vi "curvature-cator.vi"(4 "number of grid points":i32=300, 5 "decimation threshold":i32=3, 6 "first time":bool, 7 "size":i32=1, 8 "scale factor":dbl=3.0, 9 "wavepacket in":T2={"R"=0.5, "wave number"=22.0, "delta k"=7.0, "radii vector"=[], "radial section"=[], "wave vector"=22.0, "wavepacket is"=TRUE} {"delta k" format="%#_3f"; "wave number" format="%#_3f"; "R" format="%#_3f"}, 10 "z array in":cdb[](array[numeric]), 11 "omega array in":dbl[](array[numeric])) -> (1 "4 corners out":T1={"z (-pi/2)"=-1.0311345636926572+0.5736824521422934i, "z(inf)"=-0.5200164984937075+1.0975277942502903i, "z (pi/2)"=-1.0311345636926572+0.5736824521422934i, "z center"=-0.5136528600391839+0.580046090596817i, "z(0)"=-0.5200164984937075+1.0975277942502903i, "radius"=-1.0311345636926572}, 2 "spot size":dbl, 3 "spot center":cdb)   [LabVIEW 2018]
uses:
  wavepacket.ctl
  circle corners.ctl
  complex region.ctl
  <vilib>/Analysis/baseanly.llb/Median.vi
  <vilib>/Analysis/baseanly.llb/Mean.vi
  <vilib>/Analysis/baseanly.llb/Mean (DBL).vi
panel:
  out "mean":cdb
  in  "number":cdb
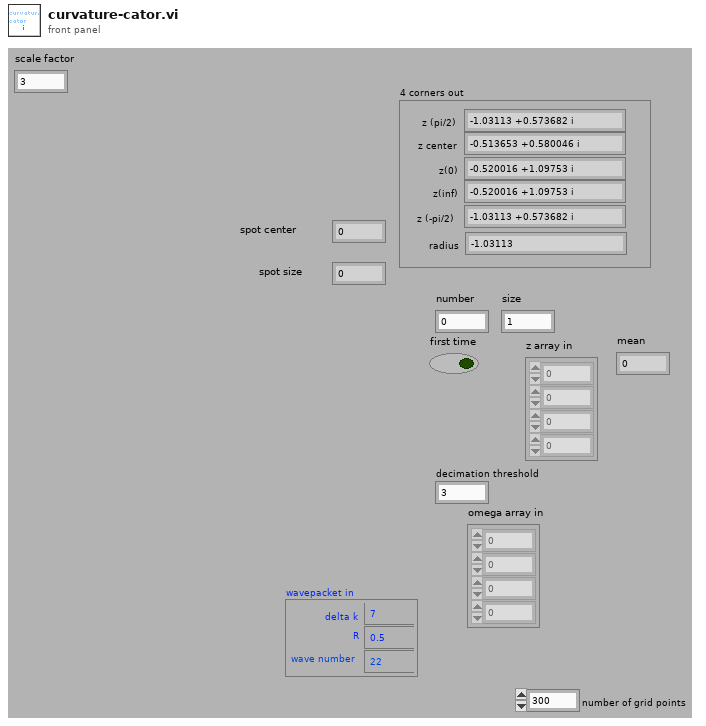
[diagram p1: front panel]
types:
  T1 = typedef "circle corners.ctl" = cluster{"z (-pi/2)":cdb, "z(inf)":cdb, "z (pi/2)":cdb, "z center":cdb, "z(0)":cdb, "radius":dbl}
  T2 = typedef "wavepacket.ctl" = cluster{"R":dbl, "wave number":dbl, "delta k":dbl, "radii vector":dbl[], "radial section":cdb[], "wave vector":dbl, "wavepacket is":bool}
  T3 = typedef "complex region.ctl" = cluster{"max re":dbl, "min re":dbl, "max im":dbl, "min im":dbl, "delta re":dbl, "delta im":dbl, "center re":dbl, "delta  z":cdb, "center im":dbl, "center z":cdb, "d im":dbl, "d re":dbl, "d z":cdb}
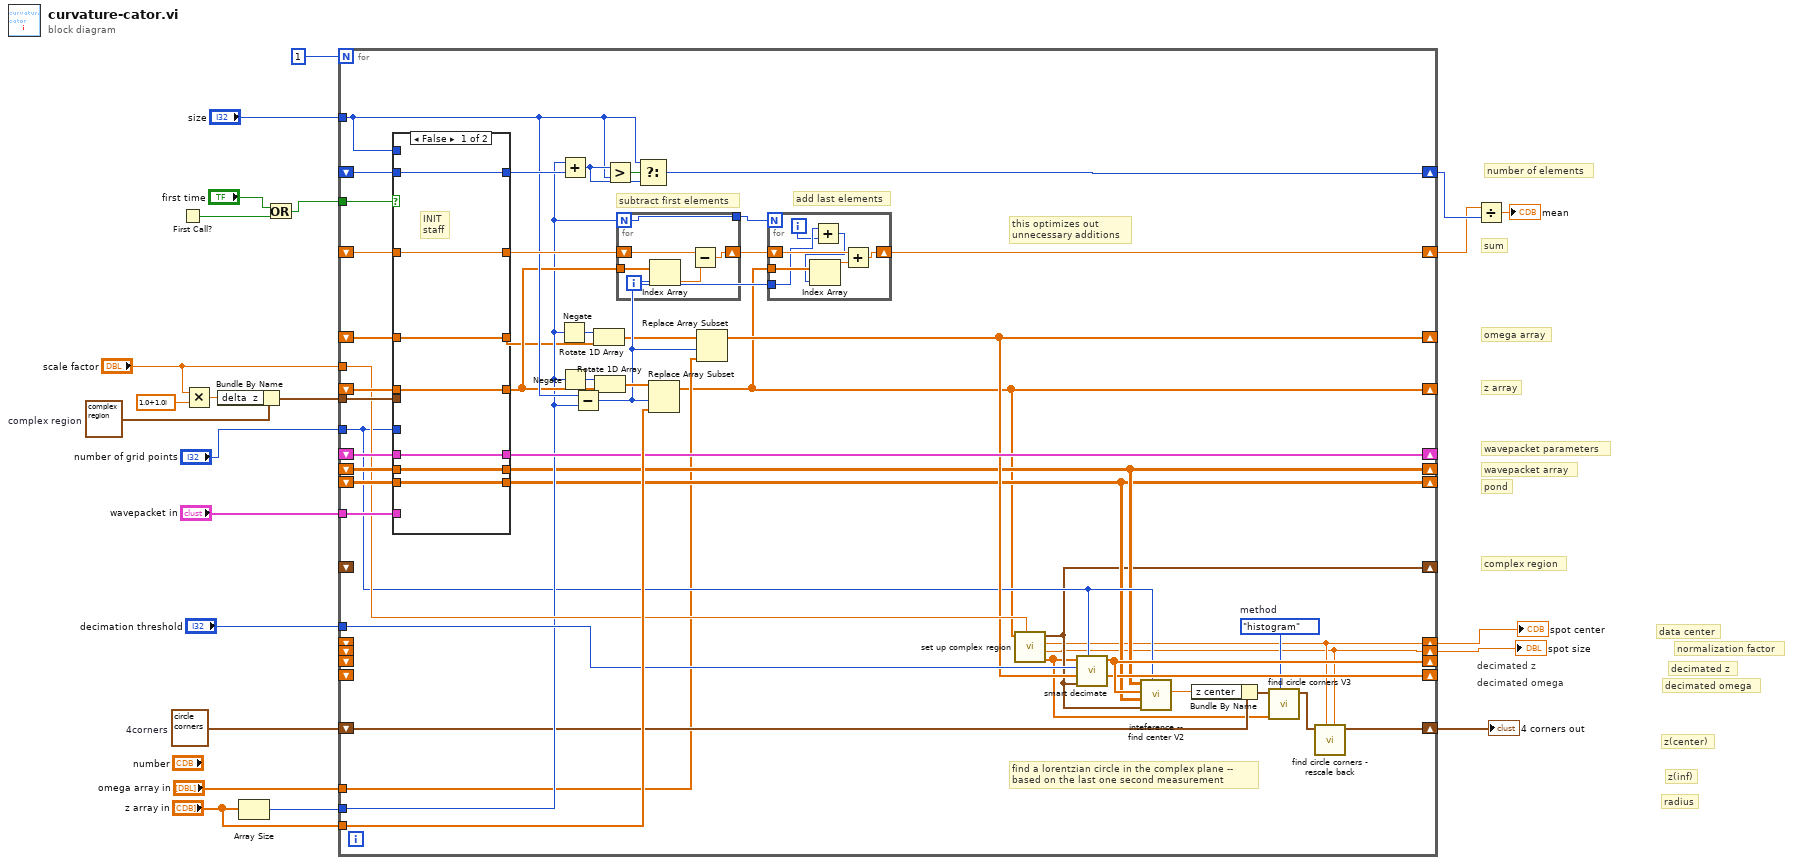
[diagram p0: block diagram]
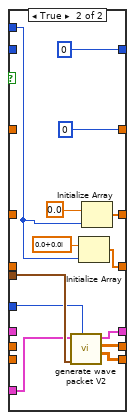
[diagram p2: hidden frame]
diagram:
  w14 = T3 {"max re"=1.5, "min re"=-1.5, "max im"=1.5, "min im"=-1.5, "delta re"=3.0, "delta im"=3.0, "center re"=0.0, "delta  z"=3.0+3.0i, "center im"=0.0, "center z"=0.0+0.0i, "d im"=0.0, "d re"=0.0, "d z"=0.0+0.0i}  # complex region
  w11 = T1 {"z (-pi/2)"=-1.0311345636926572+0.5736824521422934i, "z(inf)"=-0.5200164984937075+1.0975277942502903i, "z (pi/2)"=-1.0311345636926572+0.5736824521422934i, "z center"=-0.5136528600391839+0.580046090596817i, "z(0)"=-0.5200164984937075+1.0975277942502903i, "radius"=-1.0311345636926572}  # 4corners
  # "decimated omega"
  # "decimated z"
  # "radius"
  # "z(inf)"
  # "z(center)"
  # "decimated omega"
  # "decimated z"
  # "omega array"
  # "normalization factor"
  # "data center"
  # "pond"
  # "wavepacket array"
  # "wavepacket parameters"
  # "complex region"
  # "z array"
  # "sum"
  # "number of elements"
  n1 = First Call?() -> (First Call?: T/F=w5:bool)
  n2 = Multiply(x="scale factor", y=cdb 1.0+1.0i) -> (x*y=w1:cdb)
  n3 = Bundle By Name(cluster=w14, "delta  z"=w1) -> (w13:T3)
  n4 = Array Size(array="z array in") -> (size(s)=w19:i32)
  n5 = Or(x="first time", y=w5) -> (x .or. y?=w4:bool)
  n6 = for {
    N: 1 -> [_]
    tunnel: w4 -> [w64]
    shift-right: [w58] -> w17
    shift-left: _ -> [w69]
    shift-right: [w70] -> w21
    shift-left: _ -> [w72]
    tunnel: "size" -> [w61]
    shift-right: [w24] -> _
    shift-left: _ -> [w66]
    tunnel: w19 -> [w45]
    tunnel: "z array in" -> [w60]
    tunnel: "number of grid points" -> [w39]
    tunnel: "wavepacket in" -> [w57]
    shift-right: [w38] -> _
    shift-left: _ -> [w53]
    shift-right: [w37] -> _
    shift-left: _ -> [w52]
    shift-right: [w56] -> _
    shift-left: _ -> [w54]
    tunnel: w13 -> [w55]
    shift-right: [w36] -> _
    shift-left: _ -> [_]
    tunnel: "scale factor" -> [w50]
    shift-right: [w26] -> w9
    shift-left: _ -> [_]
    shift-right: [w25] -> w8
    shift-left: _ -> [_]
    tunnel: "decimation threshold" -> [w49]
    shift-right: [w42] -> _
    shift-left: _ -> [w48]
    shift-right: [w41] -> _
    shift-left: _ -> [_]
    shift-right: [w40] -> _
    shift-left: _ -> [_]
    shift-right: [w27] -> w7
    shift-left: w11 -> [w34]
    tunnel: "omega array in" -> [w31]
    w32 = enum16{"median", "method 2", "histogram"}."histogram"  # method
    # "find a lorentzian circle in the complex plane -- \nbased on the last one second measurement"
    # "add last elements"
    # "subtract first elements"
    # "this optimizes out \nunnecessary additions"
    n7 = case shown="False" w64 {
      tunnel: w72 -> [w92 _]
      tunnel: w69 -> [w90 _]
      tunnel: [w90 0] -> w62
      tunnel: [w92 0] -> w68
      tunnel: w66 -> [w91 _]
      tunnel: [w91 w104] -> w51
      tunnel: w61 -> [_ w100]
      tunnel: w39 -> [_ w97]
      tunnel: w57 -> [_ w96]
      tunnel: [w87 w94] -> w38
      tunnel: [w86 w93] -> w37
      tunnel: [w88 w95] -> w56
      tunnel: w55 -> [_ w98]
      tunnel: w54 -> [w88 _]
      tunnel: w53 -> [w87 _]
      tunnel: w52 -> [w86 _]
      tunnel: [w89 w99] -> w44
      tunnel: w48 -> [w89 _]
      frame False {
        # "INIT\nstaff"
      }
      frame True {
        n8 = call "generate wave packet V2.vi"("number of grid points"=w97, "complex region"=w98, "wavepacket in"=w96) -> ("pond array out"=w93:cdb[][], "wavepacket array out"=w94:cdb[][], "wavepacket out"=w95:T2)  [unwired: 6 in]
        n9 = Initialize Array(cdb 0.0+0.0i, w100) -> (w104:cdb[])
        n10 = Initialize Array(0.0, w100) -> (w99:dbl[])
      }
    }
    n11 = Negate(x=w45) -> (-x=w46:i32)
    n12 = Add(x=w45, y=w68) -> (x+y=w67:i32)
    n13 = Negate(x=w45) -> (-x=w63:i32)
    n14 = Subtract(x=w61, y=w45) -> (x-y=w47:i32)
    n15 = Rotate 1D Array(1:w44, 2:w46) -> (0:w43:dbl[])
    n16 = Rotate 1D Array(1:w51, 2:w63) -> (0:w65:cdb[])
    n17 = Greater?(x=w67, y=w61) -> (0:w71:bool)
    n18 = for {
      N: w45 -> [w80]
      tunnel: w51 -> [w84]
      shift-right: [w81] -> w59
      shift-left: w62 -> [w85]
      tunnel: [w80] -> w29
      i -> [w83]
      n19 = Index Array(array=w84, index=w83) -> (element=w82:cdb)
      n20 = Subtract(x=w85, y=w82) -> (x-y=w81:cdb)
    }
    n21 = Select(t=w61, s=w71, f=w67) -> (s? t:f=w70:i32)
    n22 = Replace Array Subset(array=w65, new element=w60, index=w47) -> (w24:cdb[])
    n23 = Replace Array Subset(array=w43, new element=w31, index=w47) -> (w42:dbl[])
    n24 = for {
      N: w29 -> [_]
      shift-right: [w77] -> w58
      shift-left: w59 -> [w79]
      tunnel: w24 -> [w76]
      tunnel: w47 -> [w74]
      i -> [w73]
      n25 = Add(x=w74, y=w73) -> (x+y=w75:i32)
      n26 = Index Array(array=w76, index=w75) -> (element=w78:cdb)
      n27 = Add(x=w79, y=w78) -> (x+y=w77:cdb)
    }
    n28 = call "set up complex region.vi"("scale factor"=w50, "z in window"=w24) -> ("z  normalized"=w30:cdb[], "normalization factor"=w25:dbl, "data center"=w26:cdb, "complex region"=w36:T3)  [unwired: 6 in]
    n29 = call "smart decimate .vi"("number of 2D grid points"=w39, "complex region"=w36, "omega in"=w42, "decimation threshold"=w49, "z in"=w30) -> ("decimated omega"=w40:dbl[], "decimated z"=w41:cdb[])  [unwired: 5 in]
    n30 = call "inteference -- find center V2.vi"("number of points"=w39, "complex region"=w36, "pond"=w37, "point sources"=w41, "wave packet"=w38) -> ("z (center)"=w35:cdb)  [unwired: 6 in]
    n31 = Bundle By Name(cluster=w34, "z center"=w35) -> (w33:T1)
    n32 = call "find circle corners V3.vi"("method"=w32, "z"=w30, "circle corners in"=w33) -> ("circle corners out"=w28:T1)  [unwired: 8 in]
    n33 = call "find circle corners - rescale back.vi"("spot size"=w25, "spot center"=w26, "4 corners in"=w28) -> ("4 corners out"=w27:T1)  [unwired: 8 in]
  }
  "spot center" <- w9
  "spot size" <- w8
  "4 corners out" <- w7
  n34 = Divide(x=w17, y=w21) -> (x/y=→"mean":cdb)
